vi "Multi Instrument Do Core.vi"(8 "error in (no error)":errorcluster, 10 "Actor in":refnum<class "Actor.lvclass">, 11 "Instrument Msg in":refnum<class "Custom Multi Instrument Msg.lvclass">) -> (0 "error out":errorcluster, 1 "Data":refnum<class "Data.lvclass">, 2 "Actor out":refnum<class "Actor.lvclass">, 3 "Instrument Msg out":refnum<class "Custom Multi Instrument Msg.lvclass">)   [LabVIEW 2020, in "Instrument Handler.lvlib" / "Custom Multi Instrument Msg.lvclass"]
doc: "Message interaction with multiple instruments is handled by the Multi Instrument Do Core.\n\nMulti Instrument Msgs contains the Cores of all the Owners they require. Keep this in mind if the message wire is branched. Incorrect synchronization of nested Multi Instrument Msgs can lead to deadlocks if wire branching is used incorrectly!\n\nThis implementaiton runs a message array and adds the resulting data to a Multi Instrument Data class."
uses:
  Custom Multi Instrument Msg.lvclass
  C:/Current projects/WS/Framework/Framework/Actors/Instrument Handler/Messages/Multi Instrument Msg/Multi Instrument Msg.lvclass
  PPL/HDH.Actor Framework.Core.Actor.lvlibp/1abvi3w/vi.lib/ActorFramework/Actor/Actor.lvclass
  PPL/HDH.Data.Generic.lvlibp/Data.lvclass
  Data/Multi Instrument Data/Multi Instrument Data.lvclass
  C:/Current projects/WS/PPL/HDH.Data.Generic.lvlibp/Data.lvclass
  Messages/Instrument Msg/Instrument Msg.lvclass
  PPL/HDH.Actor Framework.Core.Publisher.lvlibp/Messages/Response Msg/Response Msg.lvclass
  Custom Multi Instrument Msg.lvclass/Custom Multi Instrument Msg.ctl
  PPL/HDH.Actor Framework.Core.Actor.lvlibp/1abvi3w/vi.lib/ActorFramework/Message/Message.lvclass
  PPL/HDH.Actor Framework.Core.Publisher.lvlibp/Messages/Timed Msg/Data/Multi Data/Multi Data.lvclass
  Messages/Multi Instrument Msg/Multi Instrument Msg.lvclass
  C:/Current projects/WS/PPL/HDH.Actor Framework.Core.Publisher.lvlibp/Messages/Timed Msg/Data/Multi Data/Multi Data.lvclass
  C:/Current projects/WS/PPL/HDH.Actor Framework.Core.Publisher.lvlibp/Messages/Response Msg/Response Msg.lvclass
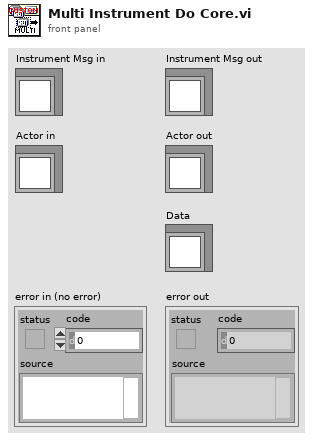
[diagram p1: front panel]
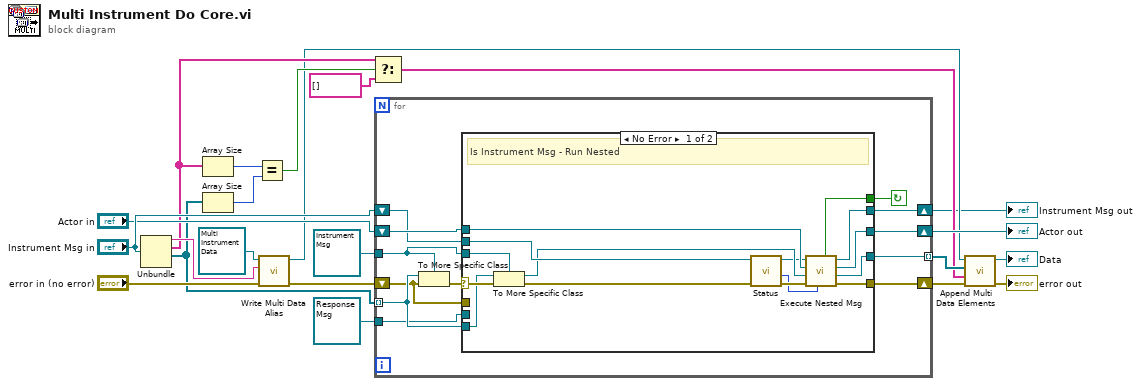
[diagram p0: block diagram]
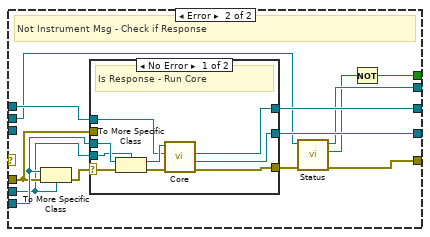
[diagram p2: hidden frame]
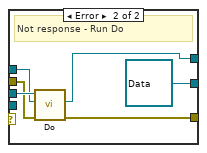
[diagram p3: hidden frame]
diagram:
  n1 = Unbundle("Instrument Msg in") -> (w21:string, w10:string[], w14:refnum<class "Message.lvclass">[])  [unwired: 1 out]
  n2 = Array Size(array=w10) -> (size(s)=w13:i32)
  n3 = Array Size(array=w14) -> (size(s)=w12:i32)
  n4 = Equal?(x=w13, y=w12) -> (x = y?=w11:bool)
  n5 = call "Write Multi Data Alias.vi"("error in (no error)"="error in (no error)", "Alias"=w21, "Multi Data in"=refnum<class "Multi Instrument Data.lvclass"> refnum ("Instrument Handler.lvlib:Multi Instrument Data.lvclass")) -> ("error out"=w15:errorcluster, "Multi Data out"=w8:refnum<class "Multi Instrument Data.lvclass">)  [unwired: 7 in]
  n6 = Select(t=w10, s=w11, f=string[] []) -> (s? t:f=w5:string[])
  n7 = for {
    tunnel: w14 -> [w28] mode=indexing
    shift-right: [w27] -> w2
    shift-left: "Instrument Msg in" -> [w31]
    tunnel: refnum<class "Instrument Msg.lvclass"> refnum ("Instrument Msg to Run") -> [w29]
    shift-right: [w33] -> w16
    shift-left: "Actor in" -> [w34]
    shift-right: [w25] -> w7
    shift-left: w15 -> [w26]
    tunnel: [w24] -> w6 mode=indexing
    tunnel: refnum<class "Response Msg.lvclass"> refnum ("HDH.Actor Framework.Core.Publisher.lvlibp:Response Msg.lvclass") -> [w23]
    stop <- w32 continue-if-true
    n8 = To More Specific Class(target class=w29, reference=w28, error in=w26) -> (error out=w30:errorcluster)  [unwired: 1 out]
    n9 = case shown="No Error" w30 {
      selector: w30 -> [w45 _]
      tunnel: w34 -> [w49 w62]
      tunnel: [w48 w61] -> w33
      tunnel: [w47 w50] -> w32
      tunnel: w31 -> [w46 w53]
      tunnel: w29 -> [w44 _]
      tunnel: w28 -> [w43 w58]
      tunnel: [w40 w52] -> w27
      tunnel: w26 -> [_ w57]
      tunnel: [w37 w54] -> w25
      tunnel: [w36 w60] -> w24
      tunnel: w23 -> [_ w56]
      frame No Error {
        # "Is Instrument Msg - Run Nested"
        n10 = To More Specific Class(target class=w44, reference=w43, error in=w45) -> (specific class reference=w42:refnum<class "Instrument Msg.lvclass">, error out=w39:errorcluster)
        n11 = call "Status.vi"("error in (no error)"=w39, "Response Msg in"=w46) -> ("error out"=w38:errorcluster, "Time to Timeout (ms)"=w35:i32, "Response Msg out"=w41:refnum<class "Custom Multi Instrument Msg.lvclass">)  [unwired: 6 in, 1 out]
        n12 = call "Execute Nested Msg.vi"("Timeout(-1ms)"=w35, "error in (no error)"=w38, "Instrument Msg to Run"=w42, "Actor in"=w49, "Multi Instrument Msg in"=w41) -> ("error out"=w37:errorcluster, "Data"=w36:refnum<class "Data.lvclass">, "Actor out"=w48:refnum<class "Actor.lvclass">, "Multi Instrument Msg out"=w40:refnum<class "Custom Multi Instrument Msg.lvclass">, "Success?"=w47:bool)  [unwired: 2 in]
      }
      frame Error {
        # "Not Instrument Msg - Check if Response"
        n13 = To More Specific Class(target class=w56, reference=w58, error in=w57) -> (error out=w59:errorcluster)  [unwired: 1 out]
        n14 = case shown="No Error" w59 {
          selector: w59 -> [w71 _]
          tunnel: w58 -> [w70 w77]
          tunnel: w62 -> [w67 w76]
          tunnel: [w66 w75] -> w61
          tunnel: [w63 w74] -> w55
          tunnel: [w65 refnum<class "Data.lvclass"> refnum ("Data")] -> w60
          tunnel: w57 -> [_ w72]
          tunnel: w56 -> [w69 _]
          frame No Error {
            # "Is Response - Run Core"
            n15 = To More Specific Class(target class=w69, reference=w70, error in=w71) -> (specific class reference=w68:refnum<class "Response Msg.lvclass">, error out=w64:errorcluster)
            n16 = call-dynamic "Core.vi"("error in (no error)"=w64, "Actor in"=w67, "Response Msg in"=w68) -> ("error out"=w63:errorcluster, "Data"=w65:refnum<class "Data.lvclass">, "Actor out"=w66:refnum<class "Actor.lvclass">)  [unwired: 5 in, 1 out]
          }
          frame Error {
            # "Not response - Run Do"
            n17 = call-dynamic "Do.vi"("error in (no error)"=w72, "Actor in"=w76, "Message"=w77) -> ("error out"=w74:errorcluster, "Actor out"=w75:refnum<class "Actor.lvclass">)  [unwired: 7 in]
          }
        }
        n18 = call "Status.vi"("error in (no error)"=w55, "Response Msg in"=w53) -> ("error out"=w54:errorcluster, "Dropped?"=w51:bool, "Response Msg out"=w52:refnum<class "Custom Multi Instrument Msg.lvclass">)  [unwired: 6 in, 1 out]
        n19 = Not(x=w51) -> (.not. x?=w50:bool)
      }
    }
  }
  "Instrument Msg out" <- w2
  "Actor out" <- w16
  n20 = call "Append Multi Data Elements.vi"("error in (no error)"=w7, "Data Alias Array"=w5, "Data Array"=w6, "Multi Data in"=w8) -> ("error out"=→"error out":errorcluster, "Multi Data out"=→"Data":refnum<class "Multi Instrument Data.lvclass">)  [unwired: 6 in]
